vi "Get Data Type.vi"(8 "error in":errorcluster, 11 "Object Entry in":refnum<class "Object Entry.lvclass">) -> (0 "error out":errorcluster, 2 "Data Type":T1=1 items=["unknown", "BOOLEAN", "INTEGER8", "INTEGER16", "INTEGER32", "UNSIGNED8", "UNSIGNED16", "UNSIGNED32", "REAL32", "VISIBLE_STRING", "OCTET_STRING", "UNICODE_STRING", "TIME_OF_DAY", "TIME_DIFFERENCE", "RESERVED1", "DOMAIN", "INTEGER24", "REAL64", "INTEGER40", "INTEGER48", "INTEGER56", "INTEGER64", "UNSIGNED24", "RESERVED2", "UNSIGNED40", "UNSIGNED48", "UNSIGNED56", "UNSIGNED64", "RESERVED3", "RESERVED4", "RESERVED5", "RESERVED6", "PDO_COMMUNICATION_PARAMETER", "PDO_MAPPING", "SDO_PARAMETER", "IDENTITY", "RESERVED7"], 3 "Object Entry out":refnum<class "Object Entry.lvclass">)   [LabVIEW 2020, in "CANopen.lvlib" / "Object Entry.lvclass"]
uses:
  Object Entry.lvclass
  Object Entry.lvclass/Object Entry.ctl
  Sub Object/Sub Object.lvclass
  Typedefs/Data Type.ctl
  CANopen.lvlib
  Sub Objects Dictionary/Sub Objects Dictionary.lvclass
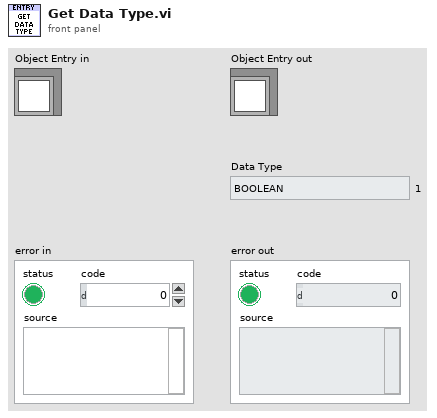
[diagram p1: front panel]
types:
  T1 = typedef "CANopen.lvlib/Data Type.ctl" = u16
  T2 = typedef "CANopen.lvlib/Object Type.ctl" = u8
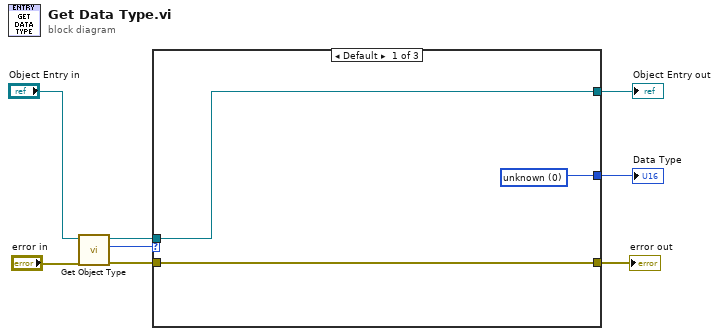
[diagram p0: block diagram]
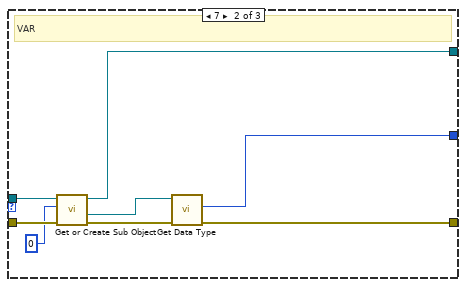
[diagram p2: hidden frame]
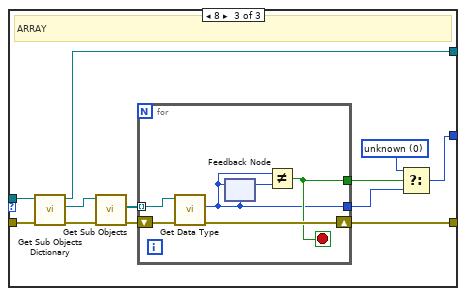
[diagram p3: hidden frame]
diagram:
  n1 = call "Get Object Type.vi"("error in"="error in", "Object Entry in"="Object Entry in") -> ("error out"=w6:errorcluster, "Object Type"=w7:T2, "Object Entry out"=w8:refnum<class "Object Entry.lvclass">)  [unwired: 7 in]
  n2 = case shown="Default" w7 {
    tunnel: w8 -> [w10 w17 w28]
    tunnel: [w10 w16 w27] -> w2
    tunnel: w6 -> [w11 w19 w29]
    tunnel: [w11 w14 w24] -> w4
    tunnel: [w9 w12 w20] -> w3
    frame Default {
      w9 = T1 0 items=["unknown", "BOOLEAN", "INTEGER8", "INTEGER16", "INTEGER32", "UNSIGNED8", "UNSIGNED16", "UNSIGNED32", "REAL32", "VISIBLE_STRING", "OCTET_STRING", "UNICODE_STRING", "TIME_OF_DAY", "TIME_DIFFERENCE", "RESERVED1", "DOMAIN", "INTEGER24", "REAL64", "INTEGER40", "INTEGER48", "INTEGER56", "INTEGER64", "UNSIGNED24", "RESERVED2", "UNSIGNED40", "UNSIGNED48", "UNSIGNED56", "UNSIGNED64", "RESERVED3", "RESERVED4", "RESERVED5", "RESERVED6", "PDO_COMMUNICATION_PARAMETER", "PDO_MAPPING", "SDO_PARAMETER", "IDENTITY", "RESERVED7"] ("Data Type")
    }
    frame 7 {
      # "VAR"
      n3 = call "Get or Create Sub Object.vi"("error in"=w19, "Sub Index"=u8 0, "Obj Entry in"=w17) -> ("error out"=w18:errorcluster, "Sub Object"=w13:refnum<class "Sub Object.lvclass">, "Obj Entry out"=w16:refnum<class "Object Entry.lvclass">)  [unwired: 6 in]
      n4 = call "Get Data Type.vi"("error in (no error)"=w18, "Sub Object in"=w13) -> ("error out"=w14:errorcluster, "Data Type"=w12:T1)  [unwired: 7 in, 1 out]
    }
    frame 8 {
      w21 = T1 0 items=["unknown", "BOOLEAN", "INTEGER8", "INTEGER16", "INTEGER32", "UNSIGNED8", "UNSIGNED16", "UNSIGNED32", "REAL32", "VISIBLE_STRING", "OCTET_STRING", "UNICODE_STRING", "TIME_OF_DAY", "TIME_DIFFERENCE", "RESERVED1", "DOMAIN", "INTEGER24", "REAL64", "INTEGER40", "INTEGER48", "INTEGER56", "INTEGER64", "UNSIGNED24", "RESERVED2", "UNSIGNED40", "UNSIGNED48", "UNSIGNED56", "UNSIGNED64", "RESERVED3", "RESERVED4", "RESERVED5", "RESERVED6", "PDO_COMMUNICATION_PARAMETER", "PDO_MAPPING", "SDO_PARAMETER", "IDENTITY", "RESERVED7"] ("t")
      # "ARRAY"
      n5 = call "Get Sub Objects Dictionary.vi"("error in"=w29, "Object Entry in"=w28) -> ("error out"=w31:errorcluster, "Sub Objects"=w30:refnum<class "Sub Objects Dictionary.lvclass">, "Object Entry out"=w27:refnum<class "Object Entry.lvclass">)  [unwired: 7 in]
      n6 = call "Get Sub Objects.vi"("error in"=w31, "Sub Objects Dictionary in"=w30) -> ("error out"=w25:errorcluster, "Sub Objects"=w26:refnum<class "Sub Object.lvclass">[])  [unwired: 7 in, 1 out]
      n7 = for {
        tunnel: w26 -> [w36] mode=indexing
        shift-right: [w35] -> w24
        shift-left: w25 -> [w37]
        tunnel: [w33] -> w23
        tunnel: [w32] -> w22
        stop <- w33 stop-if-true
        n8 = call "Get Data Type.vi"("error in (no error)"=w37, "Sub Object in"=w36) -> ("error out"=w35:errorcluster, "Data Type"=w32:T1)  [unwired: 7 in, 1 out]
        n9 = feedback-in #1(w32) -> ()
        n10 = feedback #1(w32) -> (w34:T1)
        n11 = Not Equal?(x=w32, y=w34) -> (x != y?=w33:bool)
      }
      n12 = Select(t=w21, s=w23, f=w22) -> (s? t:f=w20:T1)
    }
  }
  "error out" <- w4
  "Object Entry out" <- w2
  "Data Type" <- w3
